vi "Is equal in tolerance.vi"(4 "Absolut tolerance":dbl, 5 "Reference value":dbl, 6 "Input value":dbl) -> (0 "Is in range":bool, 2 "Coerced value":dbl)   [LabVIEW 2024]
doc: "Check if input value is in tolerance range with reference values."
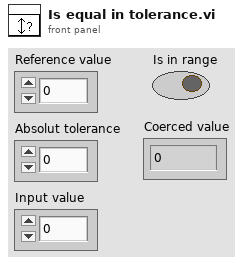
[diagram p1: front panel]
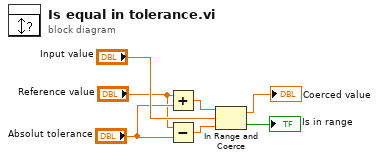
[diagram p0: block diagram]
diagram:
  n1 = Add(x="Reference value", y="Absolut tolerance") -> (x+y=w4:dbl)
  n2 = Subtract(x="Reference value", y="Absolut tolerance") -> (x-y=w3:dbl)
  n3 = In Range and Coerce(upper limit=w4, x="Input value", lower limit=w3) -> (coerced(x)=→"Coerced value":dbl, In Range?=→"Is in range":bool)
